vi "Configure Multi Eval Meas Trigger Timeout.vi"(7 "Trigger Timeout (1.00)":dbl=1.0 format="%^.3e", 8 "error in (no error)":errorcluster, 9 "Trigger Timeout Enabled (Off)":bool, 10 "Instance (1)":i32=1, 11 "VISA resource name":refnum<visa-resource-name>) -> (0 "error out":errorcluster, 3 "VISA resource name out":refnum<visa-resource-name>)   [LabVIEW 2020, in "Rohde&Schwarz CMP LR WPAN Measurement.lvlib"]
doc: "Selects the maximum time that the measurement waits for a trigger event before it stops in remote control mode or indicates a trigger timeout in manual operation mode.\n\nAttributes:\nRSCMPLRWM_ATTR_MULTIEVAL_TRIGGER_TIMEOUT\nRSCMPLRWM_ATTR_MULTIEVAL_TRIGGER_TIMEOUT_ENABLED\n\nRemote-control command:\nCONFigure:WPAN:MEAS<i>:MEValuation:TRIGger:TOUT"
uses:
  <instrlib>/Rohde&Schwarz CMP LR WPAN Measurement/Rohde&Schwarz CMP LR WPAN Measurement.lvlib
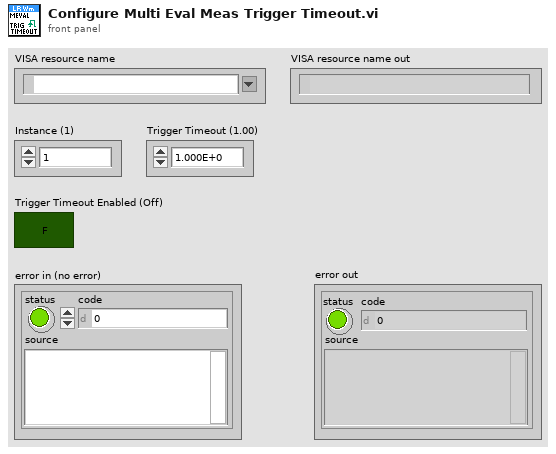
[diagram p1: front panel]
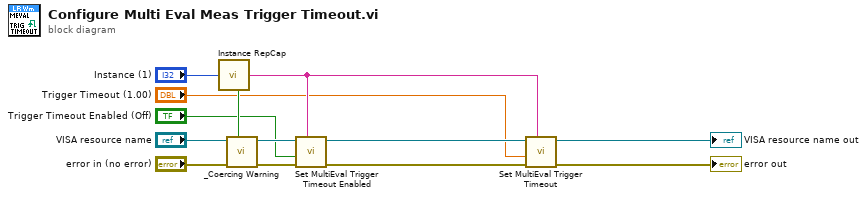
[diagram p0: block diagram]
diagram:
  n1 = call <instrlib>:"Instance RepCap.vi"("Instance In"="Instance (1)") -> ("In Range?"=w12:bool, "RepCap Identifier Out"=w13:string)  [unwired: 1 in]
  n2 = call <instrlib>:"_Coercing Warning.vi"("In Range?"=w12, "error in (no error)"="error in (no error)", "VISA resource name"="VISA resource name") -> ("error out"=w9:errorcluster, "VISA resource name out"=w8:refnum<visa-resource-name>)  [unwired: 7 in]
  n3 = call "Set MultiEval Trigger Timeout Enabled"("Repeated Capabilities"=w13, "error in (no error)"=w9, "MultiEval Trigger Timeout Enabled (OFF)"="Trigger Timeout Enabled (Off)", "instrument handle"=w8) -> ("error out"=w7:errorcluster, "instrument handle out"=w6:refnum<visa-resource-name>)  [unwired: 6 in]
  n4 = call "Set MultiEval Trigger Timeout"("Repeated Capabilities"=w13, "error in (no error)"=w7, "MultiEval Trigger Timeout (0.0)"="Trigger Timeout (1.00)", "instrument handle"=w6) -> ("error out"=→"error out":errorcluster, "instrument handle out"=→"VISA resource name out":refnum<visa-resource-name>)  [unwired: 6 in]
